vi "SetPressureUnit.vi"(11 "Device Data in":T1 {"IDS" format="%.0x"; "IDL" format="%.0x"; "IDM" format="%.0x"; "IDH" format="%.0x"}) -> (0 "Error Out":errorcluster, 1 "Message":string, 2 "Device Data out":T1 {"IDS" format="%.0x"; "IDL" format="%.0x"; "IDM" format="%.0x"; "IDH" format="%.0x"}, 3 "Function Output Comment":string)   [LabVIEW 2019]
uses:
  Device Data.ctl
  164J027_AD/Brooks DLL 1.0.1.0 32bit/Brooks DLL 1.0.1.0 Release 10032016/S Protocol/BrooksDLL.dll
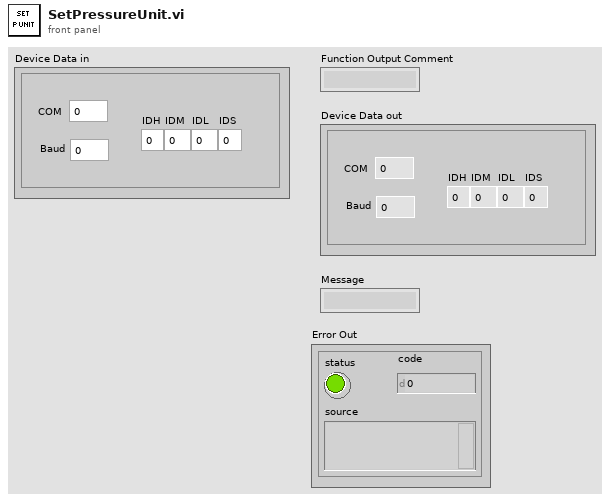
[diagram p1: front panel]
types:
  T1 = typedef "Device Data.ctl" = cluster{"COM":i32, "Baud":i32, "IDH":u8, "IDM":u8, "IDL":u8, "IDS":u8}
  T2 = cluster{bool, i32, "Function Output Comment":string}
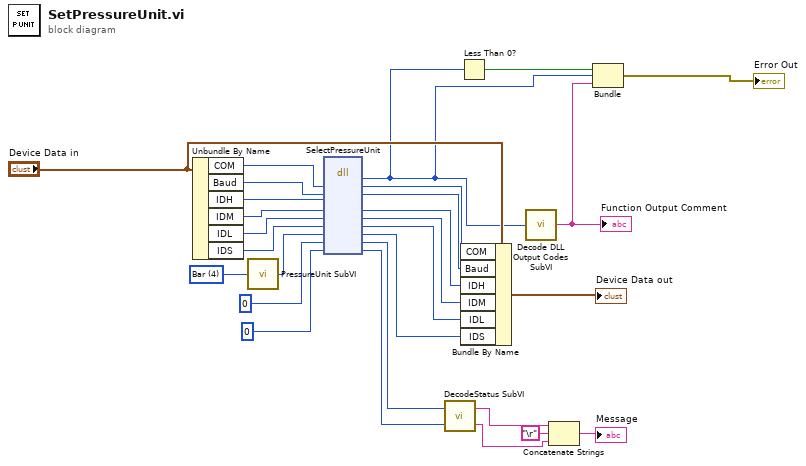
[diagram p0: block diagram]
diagram:
  w12 = u8 4 items=["In of H2O", "In of Hg", "Ft of H2O", "PSI", "Bar", "mBar", "Pascals", "kiloPascals", "Torr", "Std Atmosphere", "kg/cm2", "mTorr", "mm Hg", "gr/cm2", "cm of H2O"] ("Pressure Unit Code 2")
  n1 = Unbundle By Name("Device Data in") -> ("COM"=w15:i32, "Baud"=w16:i32, "IDH"=w20:u8, "IDM"=w19:u8, "IDL"=w18:u8, "IDS"=w17:u8)
  n2 = call "PressureUnit SubVI.vi"("Flow Unit"=w12) -> ("FlowUnit"=w13:u8)
  n3 = dll-call lib="G:/Developpement_de_Programmes/Programmes/Controle de pression/164J027_AD/Brooks DLL 1.0.1.0 32bit/Brooks DLL 1.0.1.0 Release 10032016/S Protocol/BrooksDLL.dll" fn="SelectPressureUnit"("COM"=w15, "Baud"=w16, "IDH"=w20, "IDM"=w19, "IDL"=w18, "IDS"=w17, "PressureUnitCode"=w13, "S1"=u8 0, "S2"=u8 0) -> (w3:i32, "COM"=w22:i32, "Baud"=w23:i32, "IDM"=w27:u8, "IDL"=w26:u8, "IDS"=w25:u8, "PressureUnitCode"=w24:u8, "S1"=w5:u8, "S2"=w11:u8)  [unwired: 4 in, 2 out]
  n4 = call "DecodeStatus SubVI.vi"("S2"=w11, "S1"=w5) -> ("S2 String"=w10:string, "S1 String"=w9:string)
  n5 = Less Than 0?(x=w3) -> (x < 0?=w4:bool)
  n6 = Bundle By Name(cluster="Device Data in", "COM"=w22, "Baud"=w23, "IDH"=w27, "IDM"=w26, "IDL"=w25, "IDS"=w24) -> (→"Device Data out":T1)
  n7 = call "Decode DLL Output Codes SubVI.vi"("Numeric"=w3) -> ("Function Output Comment"=w2:string)
  "Function Output Comment" <- w2
  n8 = Concatenate Strings(w9, "\r" ("string"), w10) -> (→"Message":string)
  n9 = Bundle(w4, w3, "Function Output Comment"=w2) -> (→"Error Out":T2)  [unwired: 1 in]
